vi "Deselect Platform.vi"(8 "error in (no error)":errorcluster, 11 "PlatformListPanel in":refnum<class "PlatformListPanel.lvclass">) -> (0 "error out":errorcluster, 3 "PlatformListPanel out":refnum<class "PlatformListPanel.lvclass">)   [LabVIEW 2020, in "PicoG-App.lvlib" / "PlatformListPanel.lvclass"]
uses:
  PlatformListPanel.lvclass
  PlatformListPanel.lvclass/PlatformListPanel.ctl
  PlatformArrayPanel/PlatformArrayPanel.lvclass
  <vilib>/IlluminatedG/IG OOPanel/OOPanel/ArrayManager/ArrayManager.lvclass
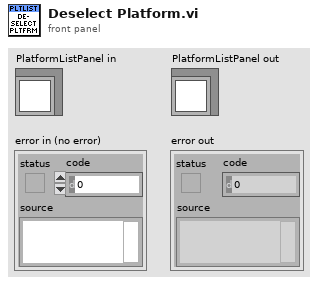
[diagram p1: front panel]
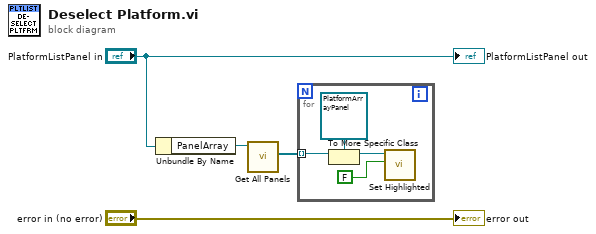
[diagram p0: block diagram]
diagram:
  n1 = Unbundle By Name("PlatformListPanel in") -> ("PanelArray"=w3:refnum<class "ArrayManager.lvclass">)
  n2 = call <vilib>:"Get All Panels.vi"("PanelArray in"=w3) -> ("Panels"=w2:refnum<class "ArrayPanel.lvclass">[])  [unwired: 8 in, 2 out]
  n3 = for {
    tunnel: w2 -> [w8] mode=indexing
    n4 = To More Specific Class(target class=refnum<class "PlatformArrayPanel.lvclass"> refnum ("PicoG-App.lvlib:PlatformArrayPanel.lvclass"), reference=w8) -> (specific class reference=w6:refnum<class "PlatformArrayPanel.lvclass">)  [unwired: 1 in, 1 out]
    n5 = call "Set Highlighted.vi"("Highlighted"=FALSE, "PlatformArrayPanel in"=w6) -> ()  [unwired: 8 in, 2 out]
  }
  "error out" <- "error in (no error)"
  "PlatformListPanel out" <- "PlatformListPanel in"
